vi "ProcAndStates.vi"(2 "FileName":string, 3 "base path":path) -> (0 "STATES":string[][](array[string]), 1 "PROCESSES":string[](array[string])=["Èíèöèàëèçàöèÿ", "ÎñòàíîâÂñåõÏðîöåññîâÈñòàðòÏðîöÈíèöèàëèçàöèÿ", "ÊîíòðîëüÄîñòîâåðíîñòè", "ÊîíòðîëüÄîñòîâåðíîñòèÎòêðûòèÿÇàòâîðàÂàêóóìíîãî", "ÊîíòðîëüÄîñòîâåðíîñòèÎòêðÇàòÂàêóóìíîãî", "ÊîíòðîëüÄîñòîâåðíîñòèÇàêðÇàòÂàêóóìíîãî", "ÊîíòðîëüÄîñòîâåðíîñòèÑîñòîÿíèÿÑàïóíà", "ÊîíòðîëüÄîñòîâåðíîñòèÑîñòîÿíèÿÓñòðîéñòâàÏëàâÏóñêà", "ÊîíòðîëüÄîñòîâåðíîñòèÑîñòîÿíèÿÏèòàíèÿÂàêóóìíîãîÍàñîñà", "ÊîíòðîëüÄîñòîâåðíîñòèÑîñòîÿíèÿÏèòàíèÿÂåíòèëÿòîðà", "ÊîíòðîëüÄîñòîâåðíîñòèÑîñòîÿíèÿÏèòàíèÿÐåãÒåìïåðàòóðû", "ÊîíòðîëüÄîñòîâåðíîñòèÑîñòîÿíèÿÏèòàíèÿÐåãÓðîâíÿ", "ÊîíòðîëüÄîñòîâåðíîñòèÓðîâíÿÂîäûÌèíèìóì", "ÊîíòðîëüÄîñòîâåðíîñòèÓðîâíÿÂîäûÌàêñèìóì", "ÊîíòðîëüÄîñòîâåðíîñòèÑîñòîÿíèÿÏèòàíèÿÍàñÎõëàæäåíèÿ", "×òåíèåÔàêòÏàðàìåòðîâ_ñ_Äàò÷èêîâ", "ÐÅÃÓËßÒÎÐ_ÒÐÀÔÈÊÀ", "×òåíèåÊîëüöåâîãîÁóôåðà", "ÎáðàáîòêàÊîìàíäÈçìåíåíèÿÍÏ_îò_ÃÓÈ", "ÎáðàáîòêàÊîìàíäÓïðàâëåíèÿ_îò_ÃÓÈ", "ÊîíòðîëüÈçìåíåíèÿ_ÔÏ_P_ÂáàêåÊîìïðåññîðà", "ÊîíòðîëüÈçìåíåíèÿ_ÔÏ_P_Âïàòðóáêå", "ÊîíòðîëüÈçìåíåíèÿ_ÔÏ_T_Âðóáàøêå", "ÊîíòðîëüÈçìåíåíèÿ_ÔÏ_T_Âáàêå", "ÊîíòðîëüÈçìåíåíèÿ_ÔÏ_P_ÂòðóáåÑèäåð", "ÊîíòðîëüÂåëè÷èíûÎòêà÷êèÂàóóìíîéÒðóáûÑèäåðîñòàòà", "ÊîíòðîëüÃîòîâíîñòèÂàêóóìà_â_Âàêóóìíîé_Òðóáå", "ÊîíòðîëüÓðîâíÿÂîäûÁàêàÎõëàæäåíèÿ", "ÊîíòðîëüÒåìïåðàòóðûÂîäûÁàêàÎõëàæäåíèÿ", "ÊîíòðîëüÒåìïåðàòóðûÐóáàøêèÎõëàæäåíèÿ", "ÊîíòðîëüÄàâëåíèÿÂáàêåÊîìïðåññîðà", "ÂÊË_ÏÈÒ_ÂÅÍÒÈËßÒÎÐ", "ÂÛÊ_ÏÈÒ_ÂÅÍÒÈËßÒÎÐ", "ÊîíòðîëüÑîñòîÿíèÿÏèòàíèÿÂåíòèëÿòîðà", "ÊîíòðîëüÑïîíòàííîãîÂûêëþ÷åíèÿÂåíòèëÿòîðà", "ÊîíòðîëüÑïîíòàííîãîÂêëþ÷åíèÿÂåíòèëÿòîðà", "ÊîíòðîëüÑîñòîÿíèÿÇàòâîðàÂàêóóìíîãî", "ÎÒÊÐ_ÇÀÒÂÎÐ_ÂÀÊ", "ÇÀÊÐ_ÇÀÒÂÎÐ_ÂÀÊ", "ÊîíòðîëüÑïîíòàííîãîÇàêðûòèÿÇàòâîðàÂàêóóìíîãî", "ÊîíòðîëüÑïîíòàííîãîÎòêðûòèÿÇàòâîðàÂàêóóìíîãî", "ÎÒÊÐ_ÑÀÏÓÍ", "ÇÀÊÐ_ÑÀÏÓÍ", "ÊîíòðîëüÑîñòîÿíèÿÏèòàíèÿÑàïóíà", "ÊîíòðîëüÑïîíòàííîãîÇàêðûòèÿÑàïóíà", "ÊîíòðîëüÑïîíòàííîãîÎòêðûòèÿÑàïóíà", "ÂÊË_ÏÈÒ_ÂÀÊ_ÍÀÑÎÑÀ", "ÂÛÊ_ÏÈÒ_ÂÀÊ_ÍÀÑÎÑÀ", "ÊîíòðîëüÑîñòîÿíèÿÏèòàíèÿÂàêóóìíîãîÍàñîñà", "ÊîíòðîëüÑïîíòàííîãîÂûêëþ÷åíèÿÂàêÍàñîñà", "ÊîíòðîëüÑïîíòàííîãîÂêëþ÷åíèÿÂàêÍàñîñà", "ÂÊË_ÏÈÒ_ÐÅÃ_Ò", "ÂÛÊ_ÏÈÒ_ÐÅÃ_Ò", "ÊîíòðîëüÑîñòîÿíèÿÏèòàíèÿÐÅÃ_Ò", "ÊîíòðîëüÑïîíòàííîãîÂûêëþ÷åíèÿÐÅÃ_Ò", "ÊîíòðîëüÑïîíòàííîãîÂêëþ÷åíèÿÐÅÃ_Ò", "ÂÊË_ÏÈÒ_ÐÅÃ_ÓÐ", "ÂÛÊ_ÏÈÒ_ÐÅÃ_ÓÐ", "ÊîíòðîëüÑîñòîÿíèÿÏèòàíèÿÐÅÃ_ÓÐ", "ÊîíòðîëüÑïîíòàííîãîÂûêëþ÷åíèÿÐÅÃ_ÓÐ", "ÊîíòðîëüÑïîíòàííîãîÂêëþ÷åíèÿÐÅÃ_ÓÐ", "ÂÊË_ÏÈÒ_ÍÀÑ_ÎÕË", "ÂÛÊ_ÏÈÒ_ÍÀÑ_ÎÕË", "ÊîíòðîëüÑîñòîÿíèÿÏèòàíèÿÍÀÑ_ÎÕË", "ÊîíòðîëüÑïîíòàííîãîÂûêëþ÷åíèÿÍàñîñàÎõëàæäåíèÿ", "ÊîíòðîëüÑïîíòàííîãîÂêëþ÷åíèÿÍàñîñàÎõëàæäåíèÿ", "ÂÊË_ÓÑÒÐ_ÏËÀÂ_ÏÓÑÊÀ", "ÂÛÊ_ÓÑÒÐ_ÏËÀÂ_ÏÓÑÊÀ", "ÊîíòðîëüÑîñòîÿíèÿÏèòàíèÿÏËÀÂ_ÏÓÑÊÀ", "ÊîíòðîëüÑïîíòàííîãîÂûêëþ÷åíèÿÏëàâíÏóñêà", "ÊîíòðîëüÑïîíòàííîãîÂêëþ÷åíèÿÏëàâíÏóñêà", "ÂÊË_ÂÀÊÓÓÌÈÐÎÂÀÍÈÅ_ÒÐÓÁÛ", "ÂÛÊ_ÂÀÊÓÓÌÈÐÎÂÀÍÈÅ_ÒÐÓÁÛ", "ÂÊË_ÂÀÊÓÓÌÍÓÞ_ÏÎÄÑÈÑÒÅÌÓ", "ÂÛÊ_ÂÀÊÓÓÌÍÓÞ_ÏÎÄÑÈÑÒÅÌÓ"])   [LabVIEW 2019]
panel:
  out "size(s)":i32[](array[numeric])=[75, 0]
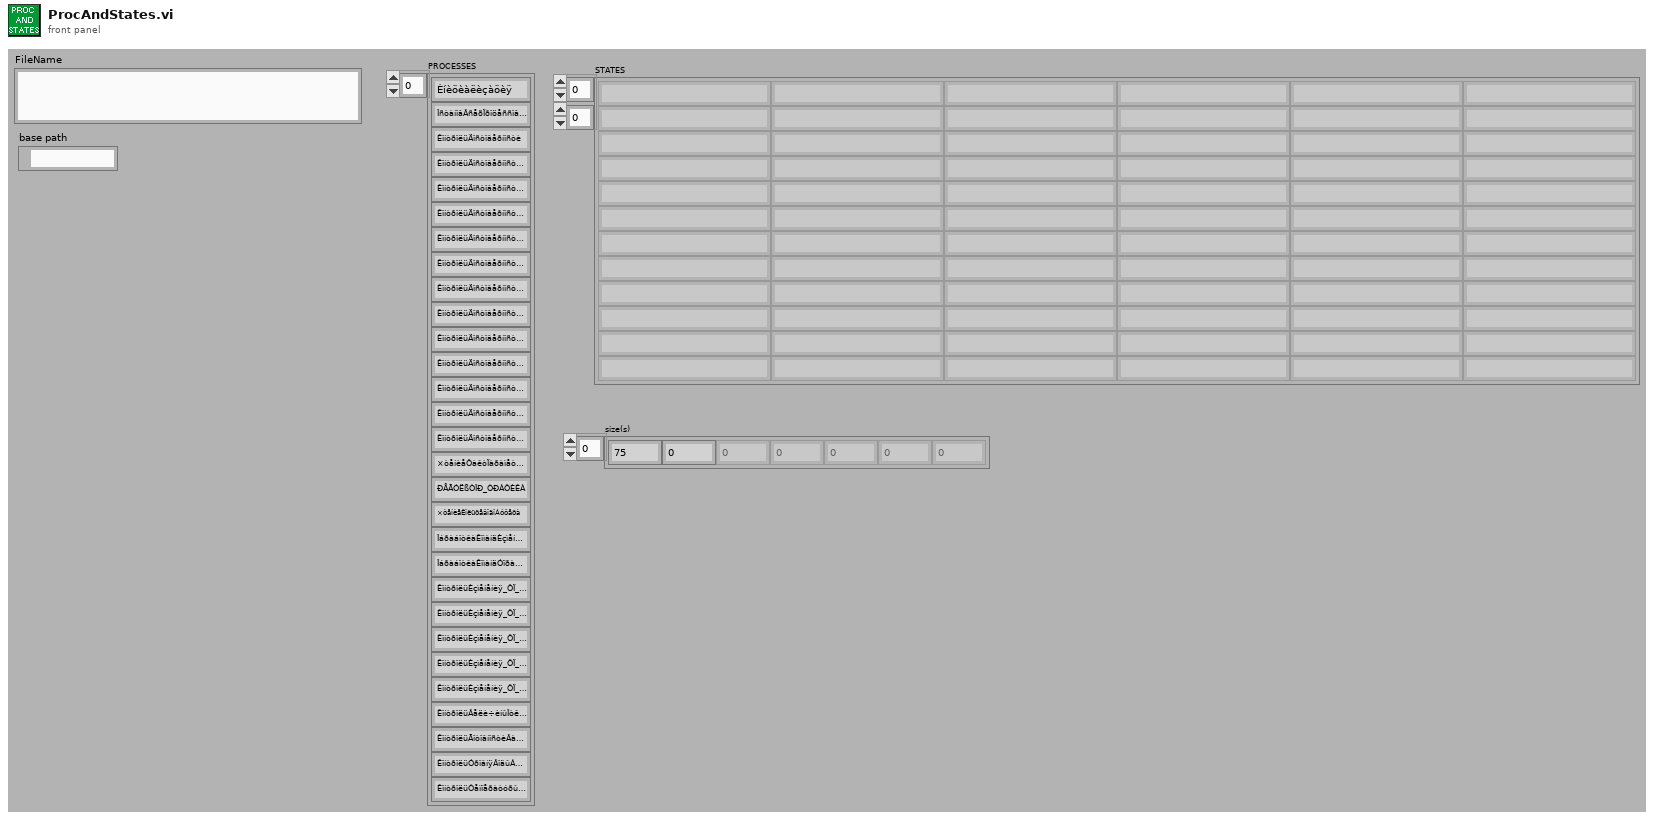
[diagram p1: front panel]
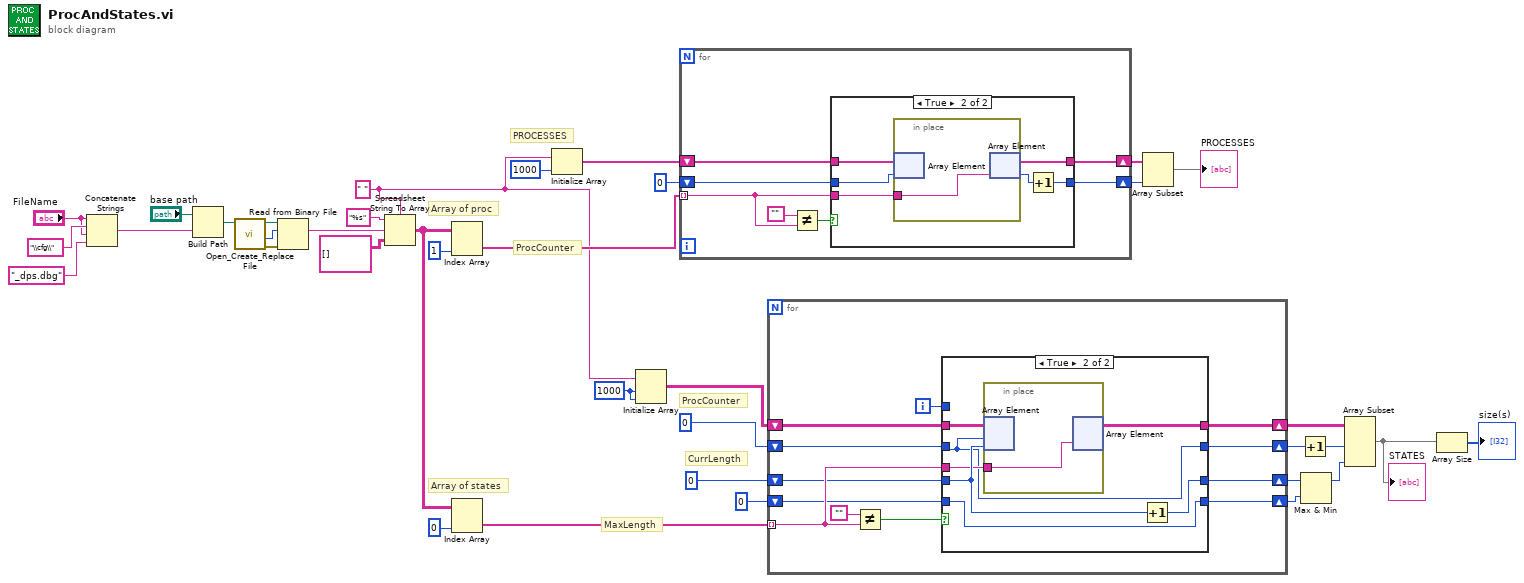
[diagram p0: block diagram]
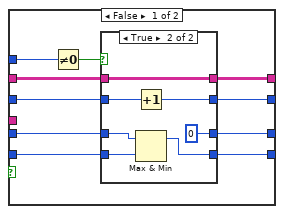
[diagram p2: hidden frame]
diagram:
  w25 = 1000 ("dimension size")
  w26 = " " ("delimiter (Tab)")
  # "ProcCounter"
  # "PROCESSES"
  # "CurrLength"
  # "MaxLength"
  # "ProcCounter"
  # "Array of proc"
  # "Array of states"
  n1 = Concatenate Strings("FileName", "\\cfg\\" ("string"), "FileName", "_dps.dbg" ("name or relative path")) -> (w3:string)
  n2 = Build Path(base path="base path", name or relative path=w3) -> (appended path=w10:path)
  n3 = call <vilib>:"Open_Create_Replace File.vi"("file path"=w10) -> ("error out"=w9:errorcluster, "file size (bytes)"=w8:i32, "refnum"=w7:refnum<file>)  [unwired: 7 in, 1 out]
  n4 = Read from Binary File(8:w9, 10:w8, 11:w7) -> (2:w1:string)  [unwired: 3 in, 3 out]
  n5 = Spreadsheet String To Array(delimiter (Tab)=w26, format string="%s", spreadsheet string=w1, array type (2D Dbl)=string[][] []) -> (array=w36:string[][])
  n6 = Index Array(array=w36, index (col)=1 ("index (row)")) -> (element=w31:string[])  [unwired: 1 in]
  n7 = Index Array(array=w36, index (col)=0 ("index (row)")) -> (element=w27:string[])  [unwired: 1 in]
  n8 = Initialize Array(w26, 1000 ("dimension size")) -> (w32:string[])
  n9 = Initialize Array(w26, w25, w25) -> (w30:string[][])
  n10 = for {
    tunnel: w31 -> [w43] mode=indexing
    shift-right: [w41] -> w19
    shift-left: w32 -> [w42]
    shift-right: [w38] -> w16
    shift-left: 0 ("dimension size") -> [w39]
    n11 = Not Equal?(x="", y=w43) -> (x != y?=w44:bool)
    n12 = case shown="True" w44 {
      tunnel: w43 -> [_ w51]
      tunnel: w42 -> [w46 w52]
      tunnel: [w46 w47] -> w41
      tunnel: w39 -> [w45 w50]
      tunnel: [w45 w48] -> w38
      frame False {
      }
      frame True {
        n13 = in-place {
          in-place-border: w51 -> [w53]
          n14 = in-place-array #1(w52, w50) -> ()  [unwired: 1 out]
          n15 = in-place-array #1(w53) -> (w47:string[], w49:i32)
        }
        n16 = Increment(x=w49) -> (x+1=w48:i32)
      }
    }
  }
  n17 = for {
    tunnel: w27 -> [w63] mode=indexing
    shift-right: [w59] -> w12
    shift-left: w30 -> [w64]
    shift-right: [w61] -> w23
    shift-left: 0 ("dimension size") -> [w62]
    shift-right: [w58] -> w21
    shift-left: 0 ("dimension size") -> [w60]
    shift-right: [w54] -> w22
    shift-left: 0 ("dimension size") -> [w55]
    i -> [w56]
    n18 = Not Equal?(x="", y=w63) -> (x != y?=w65:bool)
    n19 = case shown="True" w65 {
      tunnel: [w74 w90] -> w59
      tunnel: w64 -> [w75 w91]
      tunnel: w63 -> [_ w88]
      tunnel: w62 -> [w73 w87]
      tunnel: [w66 w87] -> w61
      tunnel: w60 -> [w72 w93]
      tunnel: [w71 w93] -> w58
      tunnel: w56 -> [w70 _]
      tunnel: w55 -> [w68 w89]
      tunnel: [w67 w92] -> w54
      frame False {
        n20 = Not Equal To 0?(x=w70) -> (x != 0?=w69:bool)
        n21 = case shown="True" w69 {
          tunnel: w75 -> [w79 w82]
          tunnel: [w79 w82] -> w74
          tunnel: w73 -> [w77 w86]
          tunnel: [w77 w81] -> w66
          tunnel: w72 -> [w78 w85]
          tunnel: [w78 w80] -> w71
          tunnel: w68 -> [w76 w84]
          tunnel: [w76 0] -> w67
          frame False {
          }
          frame True {
            n22 = Increment(x=w86) -> (x+1=w81:i32)
            n23 = Max & Min(x=w84, y=w85) -> (max(x,y)=w80:i32)  [unwired: 1 out]
          }
        }
      }
      frame True {
        n24 = in-place {
          in-place-border: w88 -> [w94]
          n25 = in-place-array #2(w91, w87, w89) -> ()  [unwired: 1 out]
          n26 = in-place-array #2(w94) -> (w90:string[][])  [unwired: 2 out]
        }
        n27 = Increment(x=w89) -> (x+1=w92:i32)
      }
    }
  }
  n28 = Array Subset(array=w19, length=w16) -> (→"PROCESSES":string[])  [unwired: 1 in]
  n29 = Increment(x=w23) -> (x+1=w11:i32)
  n30 = Max & Min(x=w22, y=w21) -> (max(x,y)=w15:i32)  [unwired: 1 out]
  n31 = Array Subset(array=w12, length (row)=w11, length (col)=w15) -> (w14:string[][])  [unwired: 2 in]
  "STATES" <- w14
  n32 = Array Size(array=w14) -> (size(s)=→"size(s)":i32[])
